vi "G#Object_GetAllObjectsFromSameOwner.vi"(1 "full class name (\"\")":string, 5 "error in (no error)":errorcluster) -> (12 "all refs":refnum<class "G#Object.lvclass">[](array[class]), 15 "external creator process owns":bool, 16 "no other owners":bool, 19 "error out":errorcluster)   [LabVIEW 2020, in "G#Object.lvclass"]
doc: "Returns all objects of the specified class with the same owner that called this method. If \"full class name\" is empty, all objects of all classes will be returned."
uses:
  G#Object.lvclass
  G#Object.lvclass/G#Object.ctl
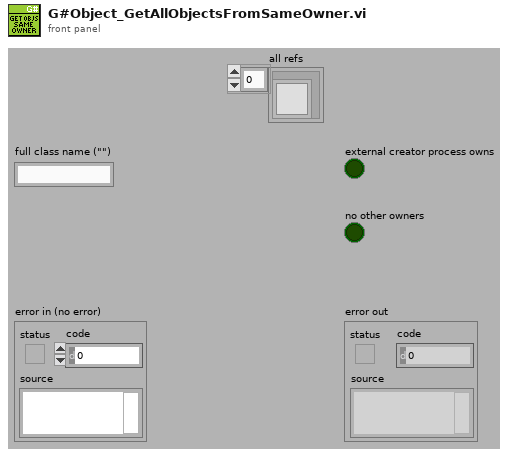
[diagram p1: front panel]
types:
  T1 = cluster{"full class name (\"\")":string, "Ref":refnum<class "G#Object.lvclass">}
  T2 = cluster{"full class name (\"\")":string, "Ref":refnum<class "G#Object.lvclass">}[]
  T3 = typedef "G#Object.lvclass/G#Object_ObjectInfoType.ctl" = cluster{"ObjectName":string, "ObjectID":u32, "Users":i32, "Counter":bool, "AttributeRefs":u32[], "FullClassName":string, "ClassName":string, "CreateMethod":T4, "GenericDestructorExists":bool, "Owner":string}
  T4 = typedef "G#Object.lvclass/G#Object_CreateMethod.ctl" = enum16{"Create", "Create or look up existing", "Look up existing"}
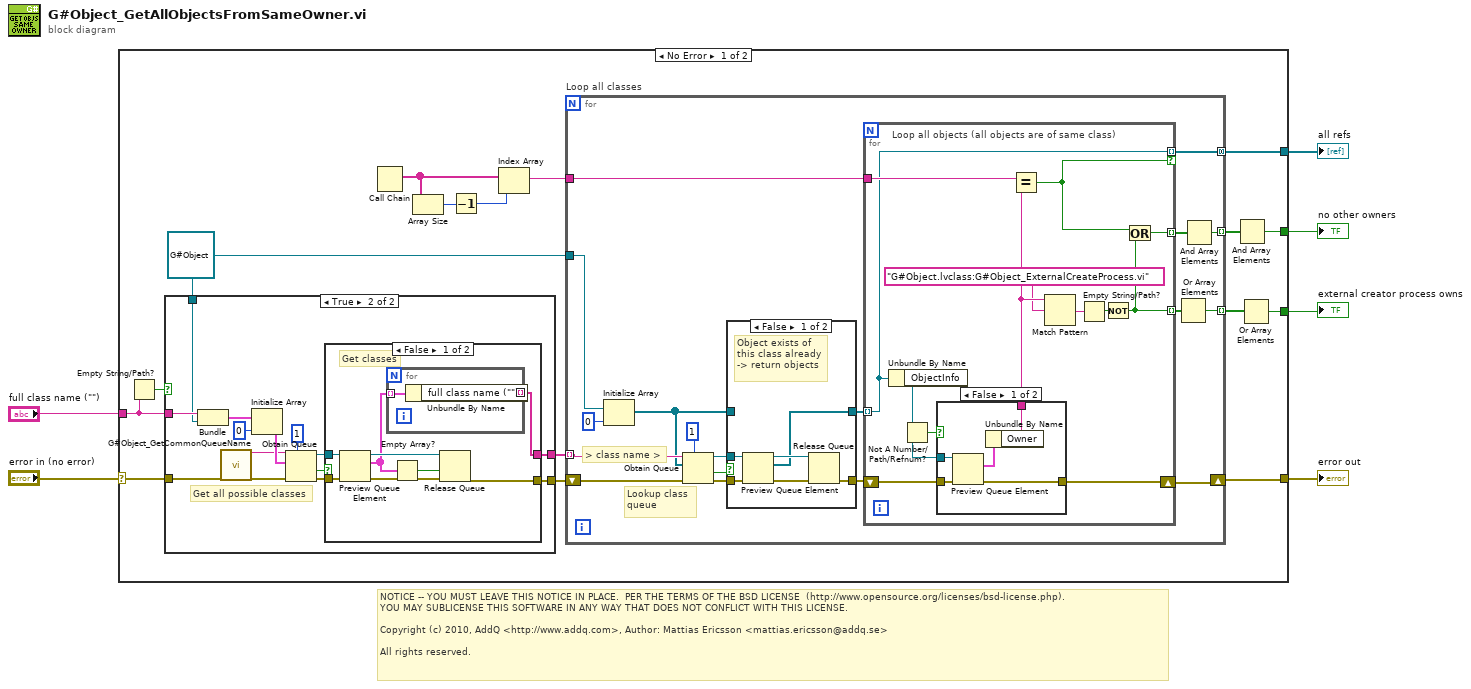
[diagram p0: block diagram]
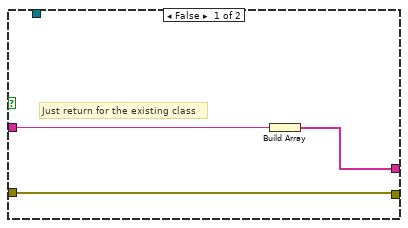
[diagram p2: hidden frame]
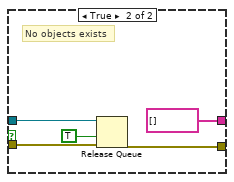
[diagram p3: hidden frame]
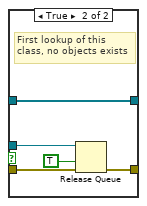
[diagram p5: hidden frame]
diagram:
  # "NOTICE -- YOU MUST LEAVE THIS NOTICE IN PLACE.  PER THE TERMS OF THE BSD LICENSE  (http://www.opensource.org/licenses/bsd-license.php).\nYOU MAY SUBLICENSE THIS SOFTWARE IN ANY WAY THAT DOES NOT CONFLICT WITH THIS LICENSE.\n\nCopyright (c) 2010, AddQ <http://www.addq.com>, Author: Mattias Ericsson <mattias.ericsson@addq.se>\n\nAll rights reserved."
  n1 = case shown="No Error" "error in (no error)" {
    selector: "error in (no error)" -> [w20 w103]
    tunnel: [w19 w103] -> w5
    tunnel: [w7 _] -> w4
    tunnel: "full class name (\"\")" -> [w17 _]
    tunnel: [w14 _] -> w2
    tunnel: [w12 _] -> w1
    frame No Error {
      w16 = refnum<class "G#Object.lvclass"> refnum ("Ref")
      n2 = Empty String/Path?(string/path=w17) -> (empty?=w18:bool)
      n3 = case shown="True" w18 {
        tunnel: [w24 w33] -> w22
        tunnel: [w25 w32] -> w21
        tunnel: w20 -> [w25 w28]
        tunnel: w17 -> [w23 w30]
        tunnel: w16 -> [_ w29]
        frame False {
          # "Just return for the existing class"
          n4 = Build Array(w23) -> (w24:string[])
        }
        frame True {
          # "Get all possible classes"
          n5 = Bundle("full class name (\"\")"=w30, "Ref"=w29) -> (w31:T1)  [unwired: 1 in]
          n6 = call "G#Object_GetCommonQueueName.vi"("error in (no error)"=w28) -> ("queue name"=w26:string, "error out"=w27:errorcluster)  [unwired: 17 in]
          n7 = Initialize Array(w31, 0 ("dimension size")) -> (w34:T2)
          n8 = Obtain Queue(max queue size (-1, unlimited)=1, name (unnamed)=w26, element data type=w34, error in (no error)=w27) -> (queue out=w37:refnum<queue>, created new?=w39:bool, error out=w38:errorcluster)  [unwired: 1 in]
          n9 = case shown="False" w39 {
            tunnel: w38 -> [w47 w51]
            tunnel: w37 -> [w46 w52]
            tunnel: [w42 string[] []] -> w33
            tunnel: [w45 w54] -> w32
            frame False {
              # "Get classes"
              n10 = Preview Queue Element(queue=w46, error in (no error)=w47) -> (queue out=w43:refnum<queue>, element=w41:T2, error out=w44:errorcluster)  [unwired: 1 in, 1 out]
              n11 = for {
                tunnel: [w49] -> w42 mode=indexing
                tunnel: w41 -> [w48] mode=indexing
                n12 = Unbundle By Name(w48) -> ("full class name (\"\")"=w49:string)
              }
              n13 = Empty Array?(array=w41) -> (empty?=w40:bool)
              n14 = Release Queue(queue=w43, force destroy? (F)=w40, error in (no error)=w44) -> (error out=w45:errorcluster)  [unwired: 2 out]
            }
            frame True {
              # "No objects exists"
              n15 = Release Queue(queue=w52, force destroy? (F)=TRUE, error in (no error)=w51) -> (error out=w54:errorcluster)  [unwired: 2 out]
            }
          }
        }
      }
      n16 = Call Chain() -> (call chain=w11:string[])
      n17 = Array Size(array=w11) -> (size(s)=w10:i32)
      n18 = Decrement(x=w10) -> (x-1=w9:i32)
      n19 = Index Array(array=w11, index=w9) -> (element=w8:string)
      n20 = for "Loop all classes" {
        shift-right: [w60] -> w19
        shift-left: w21 -> [w68]
        tunnel: w22 -> [w65] mode=indexing
        tunnel: w16 -> [w64]
        tunnel: w8 -> [w61]
        tunnel: [w58] -> w15 mode=indexing
        tunnel: [w56] -> w13 mode=indexing
        tunnel: [w55] -> w7 mode=concatenating
        # "> class name >"
        # "Lookup class\nqueue"
        n21 = Initialize Array(w64, 0 ("dimension size")) -> (w63:refnum<class "G#Object.lvclass">[])
        n22 = Obtain Queue(max queue size (-1, unlimited)=1, name (unnamed)=w65, element data type=w63, error in (no error)=w68) -> (queue out=w69:refnum<queue>, created new?=w70:bool, error out=w71:errorcluster)  [unwired: 1 in]
        n23 = case shown="False" w70 {
          tunnel: w71 -> [w96 w98]
          tunnel: w69 -> [w95 w99]
          tunnel: w63 -> [_ w102]
          tunnel: [w97 w100] -> w67
          tunnel: [w92 w102] -> w66
          frame False {
            # "Object exists of\nthis class already\n-> return objects"
            n24 = Preview Queue Element(queue=w95, error in (no error)=w96) -> (queue out=w93:refnum<queue>, element=w92:refnum<class "G#Object.lvclass">[], error out=w94:errorcluster)  [unwired: 1 in, 1 out]
            n25 = Release Queue(queue=w93, error in (no error)=w94) -> (error out=w97:errorcluster)  [unwired: 1 in, 2 out]
          }
          frame True {
            # "First lookup of this\nclass, no objects exists"
            n26 = Release Queue(queue=w99, force destroy? (F)=TRUE, error in (no error)=w98) -> (error out=w100:errorcluster)  [unwired: 2 out]
          }
        }
        n27 = for {
          shift-right: [w84] -> w60
          shift-left: w67 -> [w85]
          tunnel: w66 -> [w74] mode=indexing
          tunnel: w61 -> [w83]
          tunnel: [w82] -> w59 mode=indexing
          tunnel: [w77] -> w57 mode=indexing
          tunnel: [w74] -> w55 mode=indexing if=w73
          # "Loop all objects (all objects are of same class)"
          n28 = Unbundle By Name(w74) -> ("ObjectInfo"=w76:refnum<queue>)
          n29 = Not A Number/Path/Refnum?(number/path/refnum=w76) -> (NaN/Path/Refnum?=w75:bool)
          n30 = case shown="False" w75 {
            tunnel: w85 -> [w90 w91]
            tunnel: [w89 w91] -> w84
            tunnel: [w87 _] -> w81
            tunnel: w76 -> [w86 _]
            frame False {
              n31 = Preview Queue Element(queue=w86, error in (no error)=w90) -> (element=w88:T3, error out=w89:errorcluster)  [unwired: 1 in, 2 out]
              n32 = Unbundle By Name(w88) -> ("Owner"=w87:string)
            }
            frame True {
            }
          }
          n33 = Equal?(x=w83, y=w81) -> (x = y?=w73:bool)
          n34 = Match Pattern(string=w81, regular expression="G#Object.lvclass:G#Object_ExternalCreateProcess.vi") -> (match substring=w79:string)  [unwired: 1 in, 3 out]
          n35 = Empty String/Path?(string/path=w79) -> (empty?=w78:bool)
          n36 = Not(x=w78) -> (.not. x?=w77:bool)
          n37 = Or(x=w73, y=w77) -> (x .or. y?=w82:bool)
        }
        n38 = Or Array Elements(Boolean array=w57) -> (logical OR=w56:bool)
        n39 = And Array Elements(Boolean array=w59) -> (logical AND=w58:bool)
      }
      n40 = And Array Elements(Boolean array=w15) -> (logical AND=w14:bool)
      n41 = Or Array Elements(Boolean array=w13) -> (logical OR=w12:bool)
    }
    frame Error {
    }
  }
  "error out" <- w5
  "all refs" <- w4
  "no other owners" <- w2
  "external creator process owns" <- w1
